vi "RESTful Configure Routing Template Settings.vi"(6 "Routing Template Number (1..N)":i32, 8 "error in":errorcluster, 9 "RESTful VI routing template":T1={"Template"="", "Routing Type"=enum."Static", "HTTP Method Type"=enum."GET", "VIName"="", "Default String"="", "Require API key"=FALSE, "Auth permissions"=[], "eng_Static Alias"="", "Required Privilege"=""}, 10 "AMQP Ini In":string="#Routing Templates", 11 "Master Text In":string="#Routing Templates") -> (0 "error out":errorcluster, 2 "AMQP Ini Out":string="#Routing Templates", 3 "Master Text Out":string="#Routing Templates")   [LabVIEW 2020]
doc: "This VI configures the routing templates section of the webservices INI file."
uses:
  <vilib>/AppBuilder/AB_Classes/RESTful/AB_RESTful_RoutingTemplate.ctl
  <vilib>/AppBuilder/AB_Classes/RESTful/AB_RESTful_RoutingType.ctl
  <vilib>/AppBuilder/AB_Classes/RESTful/AB_RESTful_HTTPMethodType.ctl
  <vilib>/Utility/error.llb/whitespace.ctl
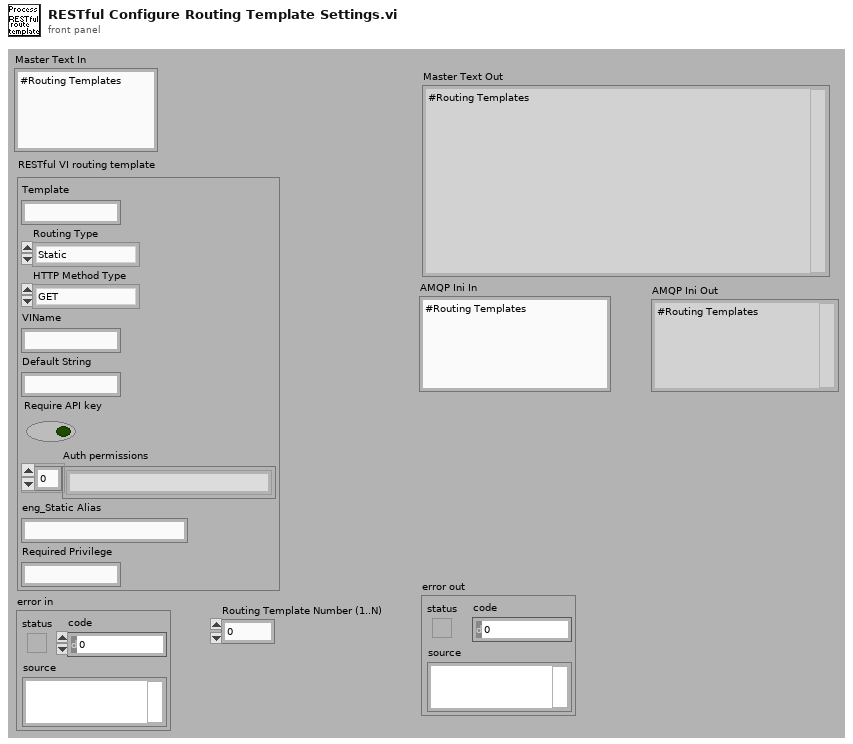
[diagram p1: front panel]
types:
  T1 = typedef "AB_RESTful_RoutingTemplate.ctl" = cluster{"Template":string, "Routing Type":T2, "HTTP Method Type":T3, "VIName":string, "Default String":string, "Require API key":bool, "Auth permissions":string[], "eng_Static Alias":string, "Required Privilege":string}
  T2 = typedef "AB_RESTful_RoutingType.ctl" = enum32{"Method", "Static"}
  T3 = typedef "AB_RESTful_HTTPMethodType.ctl" = enum32{"GET", "POST", "PUT", "DELETE"}
  T4 = typedef "whitespace.ctl" = u16
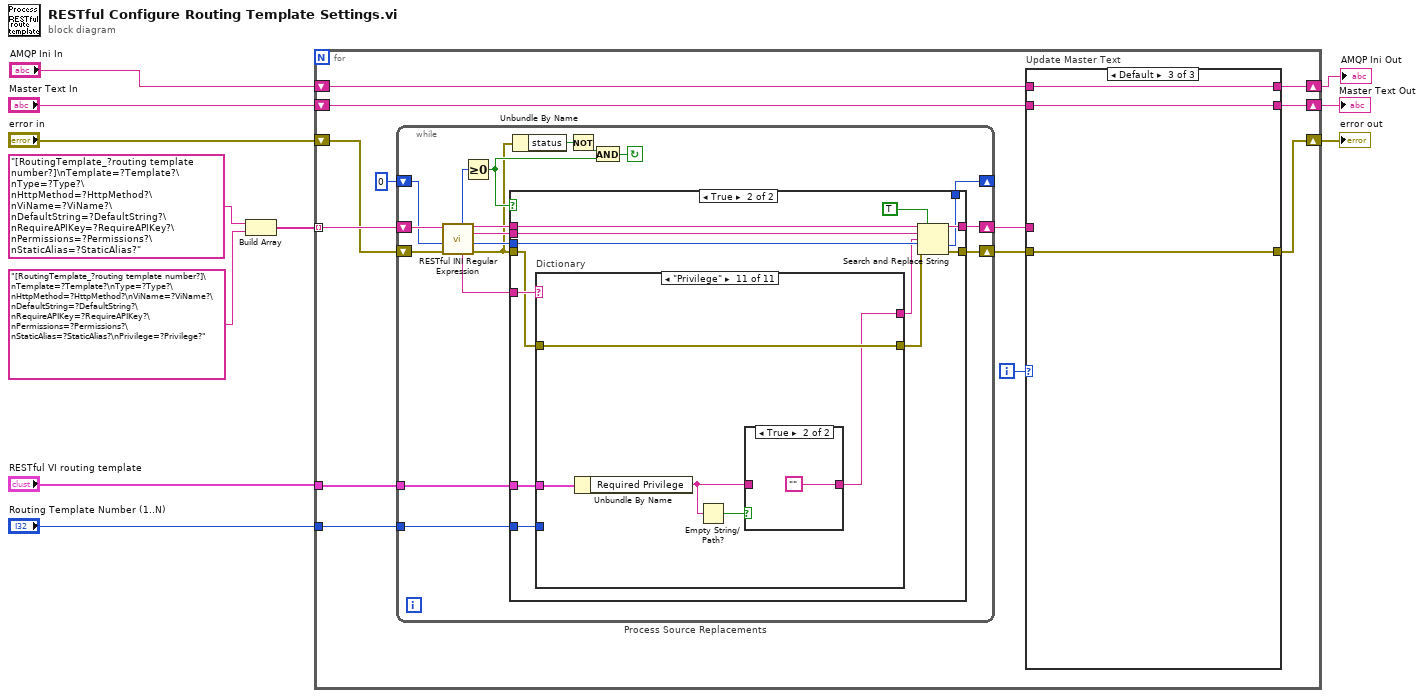
[diagram p0: block diagram]
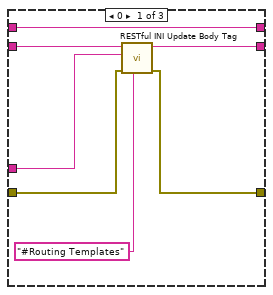
[diagram p2: hidden frame]
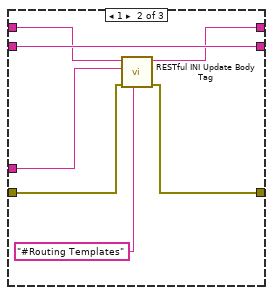
[diagram p3: hidden frame]
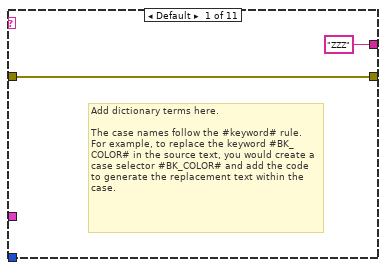
[diagram p5: hidden frame]
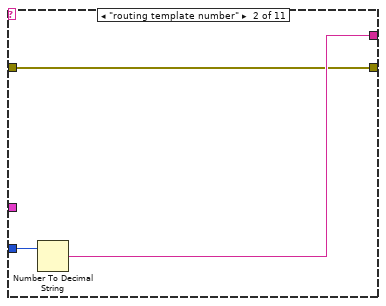
[diagram p6: hidden frame]
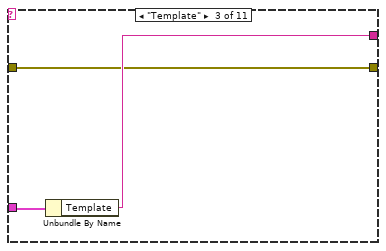
[diagram p7: hidden frame]
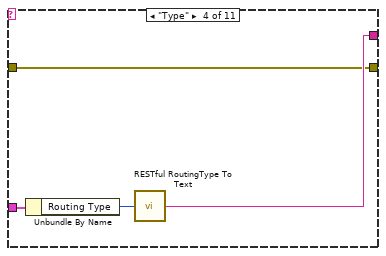
[diagram p8: hidden frame]
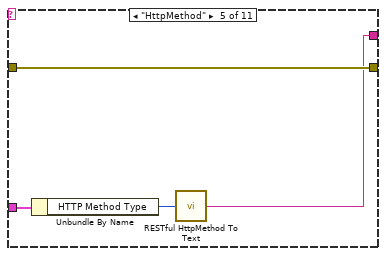
[diagram p9: hidden frame]
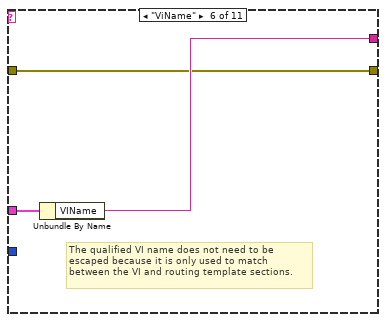
[diagram p10: hidden frame]
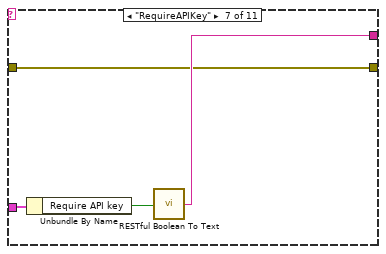
[diagram p11: hidden frame]
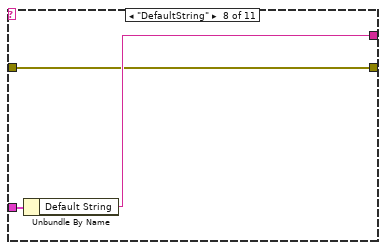
[diagram p12: hidden frame]
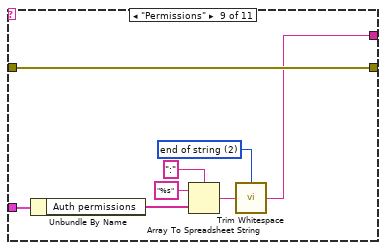
[diagram p13: hidden frame]
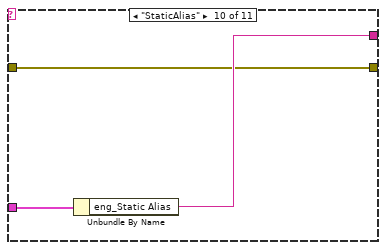
[diagram p14: hidden frame]
diagram:
  n1 = Build Array("[RoutingTemplate_?routing template number?]\nTemplate=?Template?\nType=?Type?\nHttpMethod=?HttpMethod?\nViName=?ViName?\nDefaultString=?DefaultString?\nRequireAPIKey=?RequireAPIKey?\nPermissions=?Permissions?\nStaticAlias=?StaticAlias?", "[RoutingTemplate_?routing template number?]\nTemplate=?Template?\nType=?Type?\nHttpMethod=?HttpMethod?\nViName=?ViName?\nDefaultString=?DefaultString?\nRequireAPIKey=?RequireAPIKey?\nPermissions=?Permissions?\nStaticAlias=?StaticAlias?\nPrivilege=?Privilege?") -> (w1:string[])
  n2 = for {
    tunnel: w1 -> [w24] mode=indexing
    shift-right: [w21] -> w10
    shift-left: "Master Text In" -> [w22]
    shift-right: [w18] -> w9
    shift-left: "error in" -> [w20]
    tunnel: "RESTful VI routing template" -> [w15]
    tunnel: "Routing Template Number (1..N)" -> [w14]
    shift-right: [w12] -> w5
    shift-left: "AMQP Ini In" -> [w13]
    i -> [w23]
    n3 = while "Process Source Replacements" {
      shift-right: [w54] -> w17
      shift-left: w24 -> [w59]
      shift-right: [w52] -> w19
      shift-left: w20 -> [w53]
      shift-right: [w51] -> _
      shift-left: 0 ("offset past replacement") -> [w50]
      tunnel: w15 -> [w43]
      tunnel: w14 -> [w42]
      stop <- w46 continue-if-true
      n4 = call <vilib>:"RESTful INI Regular Expression.vi"("error in"=w53, "offset (0)"=w50, "input string"=w59) -> ("error out"=w47:errorcluster, "Offset of match"=w56:i32, "whole match"=w55:string, "dup input string"=w57:string, "keyword"=w48:string, "offset past match"=w58:i32)  [unwired: 3 out]
      n5 = Greater Or Equal To 0?(x=w58) -> (x >= 0?=w49:bool)
      n6 = case shown="True" w49 {
        tunnel: w57 -> [w62 w75]
        tunnel: w56 -> [w60 w74]
        tunnel: w55 -> [_ w73]
        tunnel: [w62 w72] -> w54
        tunnel: [w61 w71] -> w52
        tunnel: w47 -> [w61 w68]
        tunnel: [w60 w70] -> w51
        tunnel: w48 -> [_ w69]
        tunnel: w43 -> [_ w66]
        tunnel: w42 -> [_ w65]
        frame False {
        }
        frame True {
          n7 = case "Dictionary" shown="\"Privilege\"" w69 {
            tunnel: w68 -> [w77 w78 w81 w84 w90 w92 w95 w99 w109 w110 w116]
            tunnel: [w77 w78 w81 w84 w90 w92 w95 w99 w109 w110 w116] -> w67
            tunnel: w66 -> [_ _ w83 w87 w91 w94 w98 w101 w108 w112 w117]
            tunnel: w65 -> [_ w80 _ _ _ _ _ _ _ _ _]
            tunnel: ["ZZZ" w79 w82 w85 w88 w93 w96 w100 w102 w111 w113] -> w64
            frame Default {
              # "Add dictionary terms here.\n\nThe case names follow the #keyword# rule.  For example, to replace the keyword #BK_COLOR# in the source text, you would create a case selector #BK_COLOR# and add the code to generate the replacement text within the case."
            }
            frame "routing template number" {
              n8 = Number To Decimal String(number=w80) -> (decimal integer string=w79:string)  [unwired: 1 out]
            }
            frame "Template" {
              n9 = Unbundle By Name(w83) -> ("Template"=w82:string)
            }
            frame "Type" {
              n10 = Unbundle By Name(w87) -> ("Routing Type"=w86:T2)
              n11 = call <vilib>:"RESTful RoutingType To Text.vi"("Routing Type"=w86) -> ("Boolean Text"=w85:string)
            }
            frame "HttpMethod" {
              n12 = Unbundle By Name(w91) -> ("HTTP Method Type"=w89:T3)
              n13 = call <vilib>:"RESTful HttpMethod To Text.vi"("HTTP Method Type"=w89) -> ("Boolean Text"=w88:string)
            }
            frame "ViName" {
              # "The qualified VI name does not need to be\nescaped because it is only used to match\nbetween the VI and routing template sections."
              n14 = Unbundle By Name(w94) -> ("VIName"=w93:string)
            }
            frame "RequireAPIKey" {
              n15 = Unbundle By Name(w98) -> ("Require API key"=w97:bool)
              n16 = call <vilib>:"RESTful Boolean To Text.vi"("Boolean"=w97) -> ("Boolean Text"=w96:string)
            }
            frame "DefaultString" {
              n17 = Unbundle By Name(w101) -> ("Default String"=w100:string)
            }
            frame "Permissions" {
              w104 = T4 2 items=["both", "start of string", "end of string"] ("location (both)")
              n18 = Unbundle By Name(w108) -> ("Auth permissions"=w103:string[])
              n19 = Array To Spreadsheet String(delimiter (Tab)=":", array=w103, 3:"%s" ("format string")) -> (spreadsheet string=w105:string)
              n20 = call <vilib>:"Trim Whitespace.vi"("string"=w105, "location (both)"=w104) -> ("trimmed string"=w102:string)
            }
            frame "StaticAlias" {
              n21 = Unbundle By Name(w112) -> ("eng_Static Alias"=w111:string)
            }
            frame "Privilege" {
              n22 = Unbundle By Name(w117) -> ("Required Privilege"=w114:string)
              n23 = Empty String/Path?(string/path=w114) -> (empty?=w115:bool)
              n24 = case shown="True" w115 {
                tunnel: [w118 ""] -> w113
                tunnel: w114 -> [w118 _]
                frame False {
                }
                frame True {
                }
              }
            }
          }
          n25 = Search and Replace String(replace all?=TRUE ("replace all? (F)"), input string=w75, search string=w73, replace string=w64, offset=w74, error in=w67) -> (result string=w72:string, offset past replacement=w70:i32, error out=w71:errorcluster)  [unwired: 3 out]
        }
      }
      n26 = Unbundle By Name(w47) -> ("status"=w45:bool)
      n27 = Not(x=w45) -> (.not. x?=w44:bool)
      n28 = And(x=w44, y=w49) -> (x .and. y?=w46:bool)
    }
    n29 = case "Update Master Text" shown="Default" w23 {
      tunnel: w22 -> [w31 w34 w41]
      tunnel: [w30 w34 w41] -> w21
      tunnel: w19 -> [w28 w37 w40]
      tunnel: [w27 w36 w40] -> w18
      tunnel: w17 -> [w29 w38 _]
      tunnel: w13 -> [w25 w33 w39]
      tunnel: [w25 w32 w39] -> w12
      frame 0 {
        n30 = call <vilib>:"RESTful INI Update Body Tag.vi"("Tag"="#Routing Templates", "error in (no error)"=w28, "Replacement String"=w29, "Input String"=w31) -> ("error out"=w27:errorcluster, "result string"=w30:string)  [unwired: 6 out]
      }
      frame 1 {
        n31 = call <vilib>:"RESTful INI Update Body Tag.vi"("Tag"="#Routing Templates", "error in (no error)"=w37, "Replacement String"=w38, "Input String"=w33) -> ("error out"=w36:errorcluster, "result string"=w32:string)  [unwired: 6 out]
      }
      frame Default {
      }
    }
  }
  "error out" <- w9
  "Master Text Out" <- w10
  "AMQP Ini Out" <- w5
